vi "ShooterSpeedRegulateV2.vi"(0 "Shooter Speed":T1(ring), 11 "Reset Shooter PID":bool) -> (4 "ALL GOOD":bool, 10 "Motor 1 Output":dbl)   [LabVIEW 2012]
uses:
  Robot Global Data.vi
  Max'sToolKit/ConvertVoltageToPercentVbs.vi
  <vilib>/addons/control/pid/NI_PID_pid.lvlib
  <vilib>/addons/control/pid/pid.llb/PID (DBL).vi
panel:
  out "Loop Rate (Hz)":dbl
  out "Array Index":dbl
  out "Wheel 1 RPS":dbl
  out "W1 Target RPS":dbl
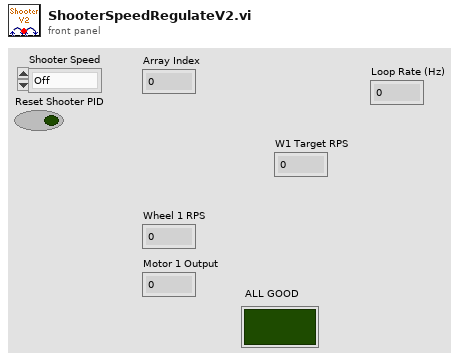
[diagram p1: front panel]
types:
  T1 = enum16{"Off", "Close Pyramid 3pt", "Far Pyramid 3pt", "Feeder Shot"}
  T2 = typedef "WPI_EncoderDevRef.ctl" = cluster{"DevStatus":errorcluster, "EncoderIndex":T3, "CounterIndex":T4, "DistancePerCount":dbl, "Decoding Type":T5}
  T3 = typedef "FPGA_EncoderIdx.ctl" = enum8{"Enc 0", "Enc 1", "Enc 2", "Enc 3", "Invalid"}
  T4 = typedef "FPGA_CounterCtrSystemIndex.ctl" = enum8{"Ctr 0", "Ctr 1", "Ctr 2", "Ctr 3", "Ctr 4", "Ctr 5", "Ctr 6", "Ctr 7", "Invalid"}
  T5 = typedef "WPI_EncoderType.ctl" = enum16{"1x", "2x", "4x"}
  T6 = cluster{"Target Voltage":dbl, "Target Speed":dbl, "Angle Up?":bool}[]
  T7 = cluster{"Target Voltage":dbl, "Target Speed":dbl, "Angle Up?":bool}
  T8 = cluster{"proportional gain (Kc)":dbl, "integral time (Ti, min)":dbl, "derivative time (Td, min)":dbl}
  T9 = typedef "WPI_MotorControlDeviceRef.ctl" = cluster{"DeviceStatus":errorcluster, "Type":enum16{"PWM", "CAN"}, "PWM":cluster{"Digital Module":T10, "PWM Channel":T11, "DeadBand":T12}, "CAN":cluster{"Device Number":u8, "Control Mode":T13, "Semaphore":T14, "Max Vout":dbl}, "Invert":bool, "TransformRef":T15, "InvTransformRef":T15}
  T10 = typedef "FPGA_TypedefDigitalModule.ctl" = enum16{"Digital Module 1", "Digital Module 2"}
  T11 = typedef "FPGA_DIOPWMChannel.ctl" = enum8{"PWM 1", "PWM 2", "PWM 3", "PWM 4", "PWM 5", "PWM 6", "PWM 7", "PWM 8", "PWM 9", "PWM 10", "Invalid"}
  T12 = typedef "WPI_PWMDeadband.ctl" = cluster{"Name":string, "maxPositivePwm":i32, "minPositivePwm":i32, "centerPwm":i32, "maxNegativePwm":i32, "minNegativePwm":i32, "angularRange":u16}
  T13 = typedef "WPI_CANJaguar_ControlMode.ctl" = enum8{"Percent VBus", "Current", "Speed", "Position", "Voltage"}
  T14 = typedef "Semaphore RefNum" = refnum<k1>
  T15 = typedef "WPI_PWMTransform_ConPane.ctl" = refnum<vi>
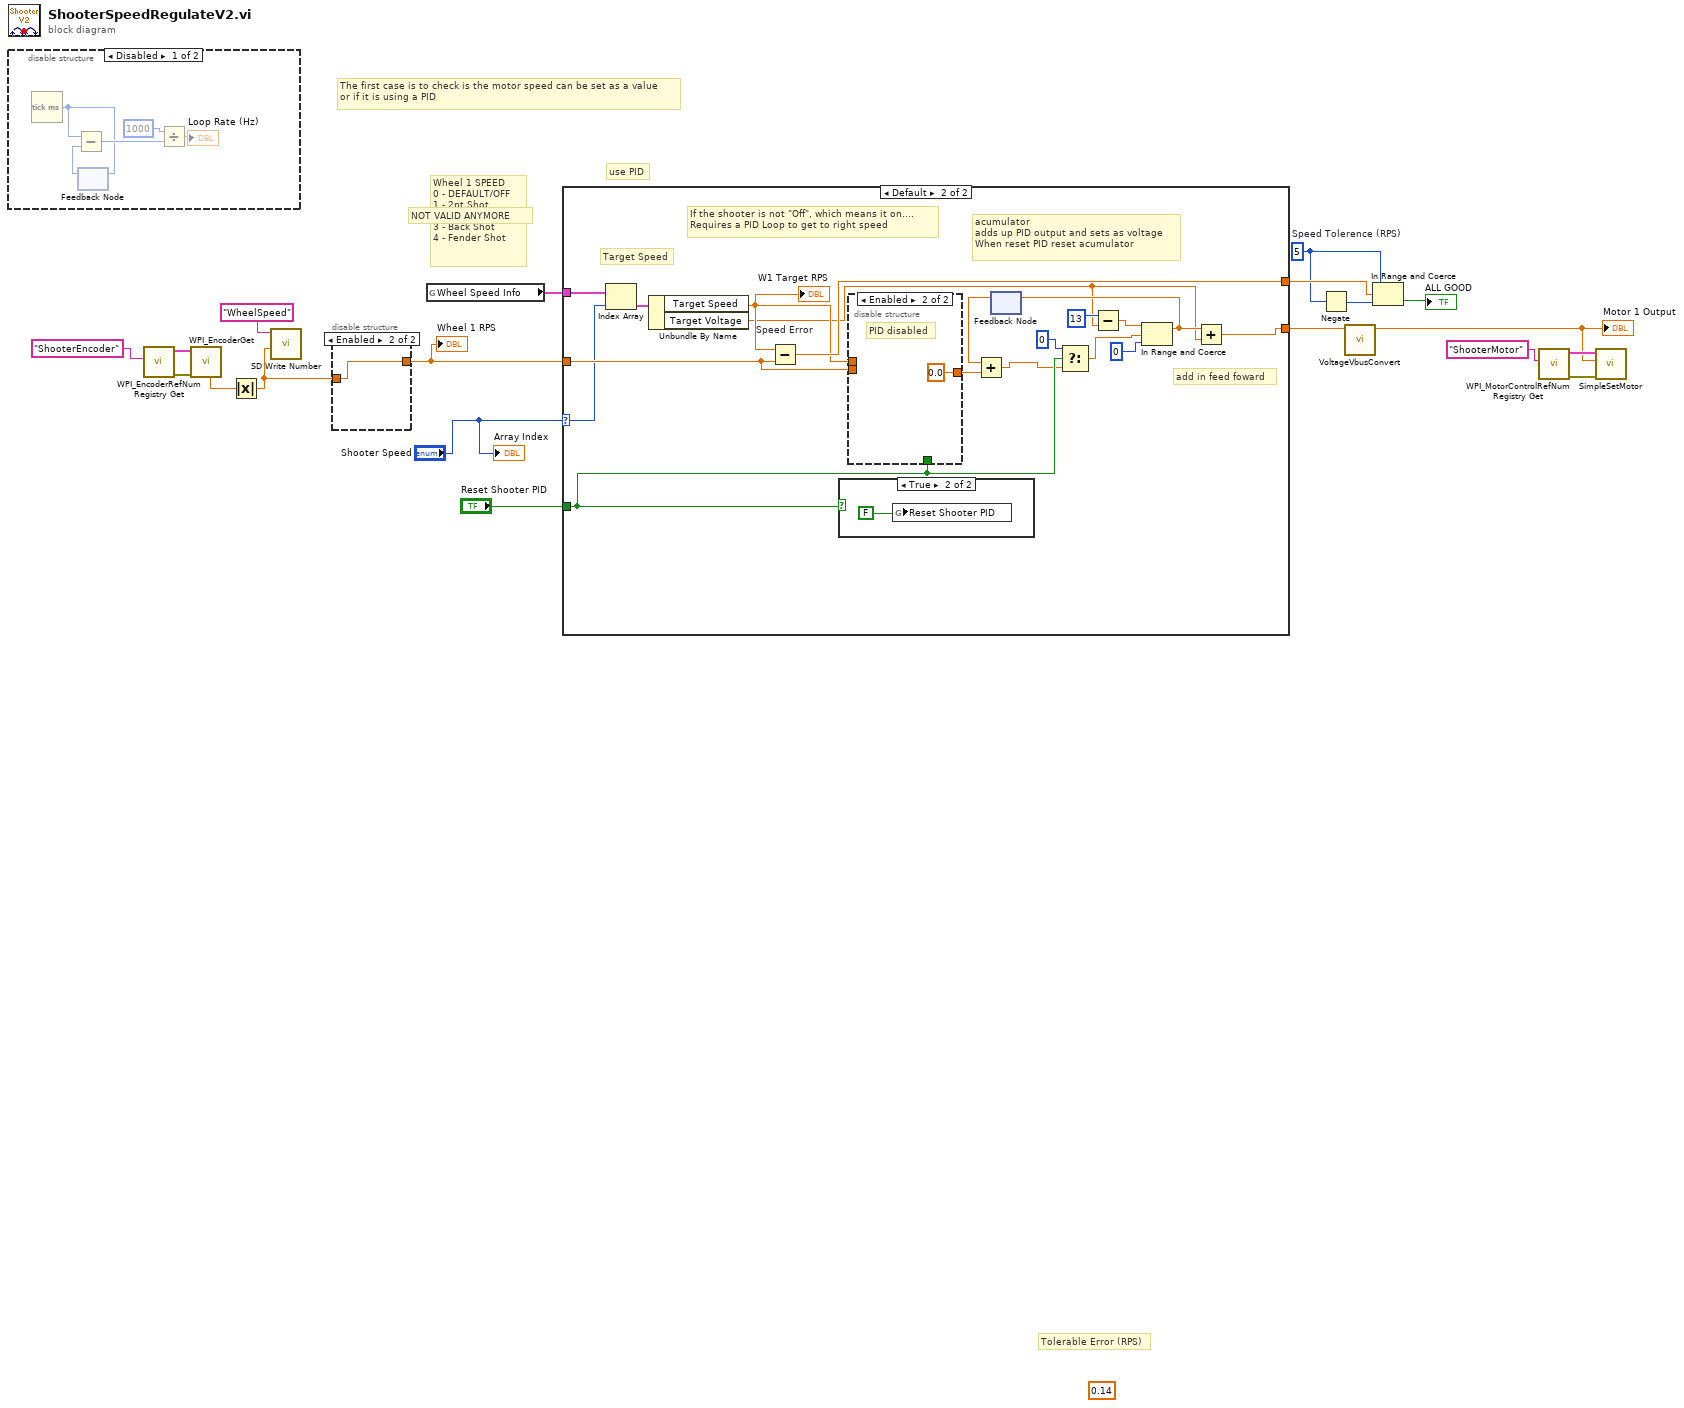
[diagram p0: block diagram]
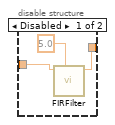
[diagram p2: hidden frame]
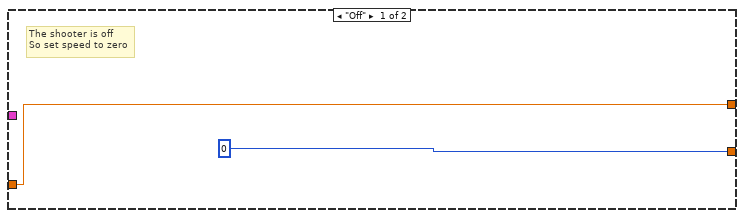
[diagram p4: hidden frame]
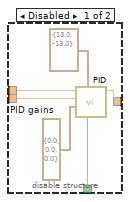
[diagram p5: hidden frame]
diagram:
  w6 = 5  # Speed Tolerence (RPS)
  (unwired) 0.14
  # "use PID"
  # "NOT VALID ANYMORE"
  # "The first case is to check is the motor speed can be set as a value\nor if it is using a PID"
  # "Tolerable Error (RPS)"
  # "Wheel 1 SPEED\n0 - DEFAULT/OFF\n1 - 2pt Shot\n2 - 3pt Key Shot\n3 - Back Shot\n4 - Fender Shot"
  n1 = disable-structure shown="Disabled" {
    frame Disabled {
      n2 = Tick Count (ms)() -> (millisecond timer value=w20:u32)
      n3 = feedback #1() -> (w21:u32)  [unwired: 1 in]
      n4 = Subtract(x=w20, y=w21) -> (x-y=w23:u32)
      n5 = feedback-in #1(w20) -> ()
      n6 = Divide(x=1000, y=w23) -> (x/y=→"Loop Rate (Hz)":dbl)
    }
    frame Enabled {
    }
  }
  n7 = call <vilib>:"WPI_EncoderRefNum Registry Get.vi"("refnum name"="ShooterEncoder") -> ("error out"=w12:errorcluster, "EncoderDevRef"=w13:T2)  [unwired: 9 in]
  n8 = call <vilib>:"WPI_EncoderGet.vi"("error in (no error)"=w12, "EncoderDevRef"=w13) -> ("Rate"=w9:dbl)  [unwired: 4 in, 5 out]
  n9 = Absolute Value(x=w9) -> (abs(x)=w2:dbl)
  n10 = call <vilib>:"SD Write Number.vi"("Numeric"=w2, "Name"="WheelSpeed") -> ()  [unwired: 8 in, 2 out]
  n11 = disable-structure shown="Enabled" {
    disable-tunnel: [w26 w28] -> w11
    disable-tunnel: w2 -> [w25 w28]
    frame Disabled {
      n12 = call "FIRFilter.vi"("Filter Size"=5.0 ("Filter size"), "Input"=w25) -> ("Output"=w26:dbl)  [unwired: 9 in]
    }
    frame Enabled {
    }
  }
  "Wheel 1 RPS" <- w11
  n13 = global read "Robot Global Data.vi" "Wheel Speed Info"() -> (w10:T6)
  n14 = case shown="Default" "Shooter Speed" {
    selector: "Shooter Speed" -> [_ w40]
    tunnel: w11 -> [w29 w46]
    tunnel: [0 w37] -> w5
    tunnel: [w29 w47] -> w15
    tunnel: w10 -> [_ w44]
    tunnel: "Reset Shooter PID" -> [_ w42]
    frame "Off" {
      # "The shooter is off\nSo set speed to zero"
    }
    frame Default {
      # "add in feed foward"
      # "acumulator\nadds up PID output and sets as voltage\nWhen reset PID reset acumulator"
      # "Target Speed"
      # "If the shooter is not \"Off\", which means it on....\nRequires a PID Loop to get to right speed"
      n15 = Index Array(array=w44, index=w40) -> (element=w33:T7)
      n16 = Unbundle By Name(w33) -> ("Target Speed"=w32:dbl, "Target Voltage"=w31:dbl)
      "W1 Target RPS" <- w32
      n17 = Subtract "Speed Error"(x=w32, y=w46) -> (x-y=w47:dbl)
      n18 = case shown="True" w42 {
        frame False {
        }
        frame True {
          n19 = global write "Robot Global Data.vi" "Reset Shooter PID"(FALSE) -> ()
        }
      }
      n20 = disable-structure shown="Enabled" {
        disable-tunnel: w46 -> [w52 _]
        disable-tunnel: w32 -> [w51 _]
        disable-tunnel: w42 -> [w50 _]
        disable-tunnel: [w49 0.0 ("output")] -> w41
        frame Disabled {
          w53 = T8 {"proportional gain (Kc)"=0.0, "integral time (Ti, min)"=0.0, "derivative time (Td, min)"=0.0}  # PID gains
          n21 = call-poly <vilib>:"PID.vi"("reinitialize? (F)"=w50, "output range"=cluster{"output high":dbl, "output low":dbl} {"output high"=13.0, "output low"=-13.0}, "PID gains"=w53, "process variable"=w52, "setpoint"=w51) -> ("output"=w49:dbl)  [unwired: 5 in, 1 out]
        }
        frame Enabled {
          # "PID disabled"
        }
      }
      n22 = feedback #2() -> (w43:dbl)  [unwired: 1 in]
      n23 = Add(x=w43, y=w41) -> (x+y=w36:dbl)
      n24 = Select(t=0, s=w42, f=w36) -> (s? t:f=w39:dbl)
      n25 = Subtract(x=13 ("upper limit"), y=w31) -> (x-y=w34:dbl)
      n26 = In Range and Coerce(upper limit=w34, x=w39, lower limit=0 ("upper limit")) -> (coerced(x)=w38:dbl)  [unwired: 1 out]
      n27 = feedback-in #2(w38) -> ()
      n28 = Add(x=w38, y=w31) -> (x+y=w37:dbl)
    }
  }
  n29 = Negate(x=w6) -> (-x=w16:i32)
  n30 = call-poly "VoltageVbusConvert.vi"("Voltage"=w5) -> ("Vbus"=w4:dbl)  [unwired: 10 in]
  "Motor 1 Output" <- w4
  n31 = In Range and Coerce(upper limit=w6, x=w15, lower limit=w16) -> (In Range?=→"ALL GOOD":bool)  [unwired: 1 out]
  n32 = call <vilib>:"WPI_MotorControlRefNum Registry Get.vi"("refnum name"="ShooterMotor") -> ("error out"=w17:errorcluster, "MotorControlDevRef"=w18:T9)  [unwired: 9 in]
  n33 = call "SimpleSetMotor.vi"("error in (no error)"=w17, "Output"=w4, "MotorControlDevRef"=w18) -> ()  [unwired: 7 in, 2 out]
  "Array Index" <- "Shooter Speed"
